vi "GetApplicationPaths.vi"(8 "error in (no error)":errorcluster) -> (0 "error out":errorcluster, 3 "ApplicationPath":T1)   [LabVIEW 2013]
uses:
  Ctrls/ApplicationPaths.ctl
  Ctrls/EnumFgvConfigCommand.ctl
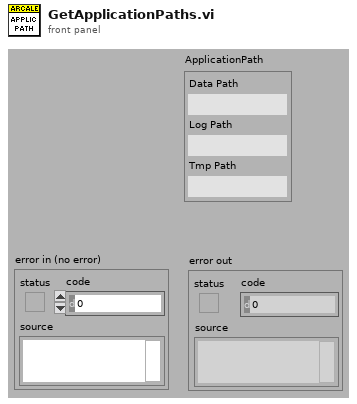
[diagram p1: front panel]
types:
  T1 = typedef "ApplicationPaths.ctl" = cluster{"Data Path":path, "Log Path":path, "Tmp Path":path}
  T2 = typedef "EnumFgvConfigCommand.ctl" = enum16{"Load", "Get", "Set", "Save To Disk"}
  T3 = typedef "ApplicationConfig.ctl" = cluster{"Data Path":path, "MessageHandlerConfig":T4, "Simulation":bool, "Dictionnary":string}
  T4 = typedef "MessageHandlerConfig.ctl" = cluster{"Max log files":u32, "Max messages per file":u32}
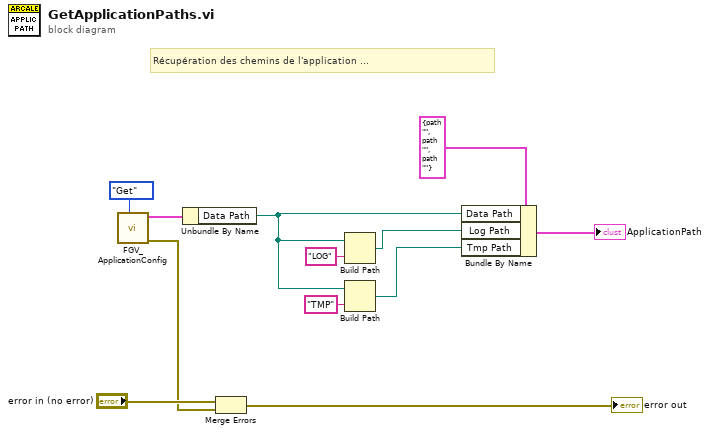
[diagram p0: block diagram]
diagram:
  # "Récupération des chemins de l'application ..."
  n1 = call "FGV_ApplicationConfig.vi"("Command"=EnumFgvConfigCommand."Get") -> ("error out"=w4:errorcluster, "ApplicationConfigOut"=w11:T3)  [unwired: 9 in]
  n2 = Unbundle By Name(w11) -> ("Data Path"=w1:path)
  n3 = Merge Errors("error in (no error)", w4) -> (→"error out":errorcluster)
  n4 = Build Path(base path=w1, name or relative path="LOG") -> (appended path=w6:path)
  n5 = Build Path(base path=w1, name or relative path="TMP") -> (appended path=w2:path)
  n6 = Bundle By Name(cluster=T1 {"Data Path"=path "", "Log Path"=path "", "Tmp Path"=path ""} ("ApplicationPath"), "Data Path"=w1, "Log Path"=w6, "Tmp Path"=w2) -> (→"ApplicationPath":T1)
